vi "Rundenzeit.vi"(11 "Startlinie":bool) -> (3 "Rundenzeiten":dbl[](array[numeric])=[inf, inf, inf, inf, inf, inf, inf])   [LabVIEW 2016]
panel:
  # "Minimum"
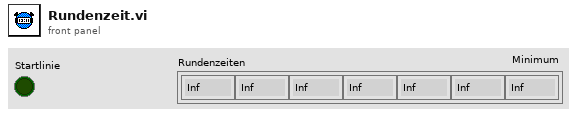
[diagram p1: front panel]
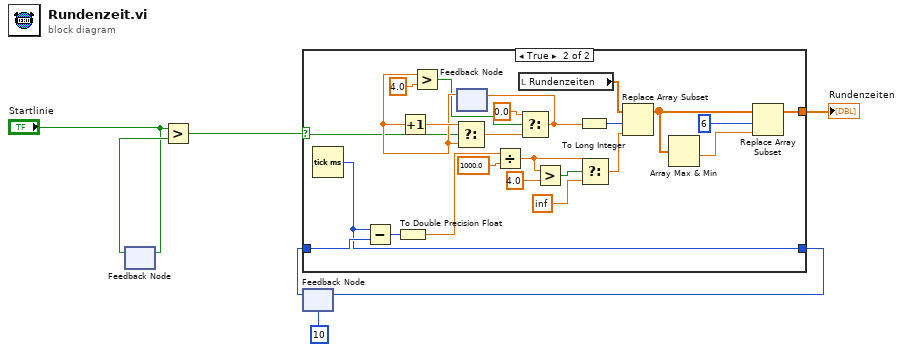
[diagram p0: block diagram]
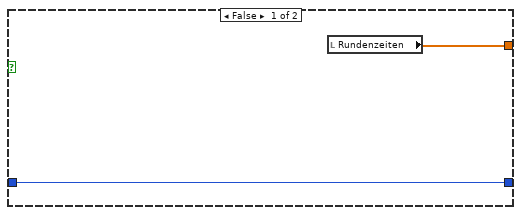
[diagram p2: hidden frame]
diagram:
  n1 = feedback #1() -> (w5:bool)  [unwired: 1 in]
  n2 = feedback-in #1("Startlinie") -> ()
  n3 = Greater?(x="Startlinie", y=w5) -> (0:w1:bool)
  n4 = feedback #2(u32 10 ("millisecond timer value")) -> (w6:u32)
  n5 = case shown="True" w1 {
    selector: w1 -> [_ w23]
    tunnel: [w9 w30] -> w7
    tunnel: w6 -> [w9 w33]
    tunnel: [w8 w19] -> w3
    frame False {
      n6 = local read "Rundenzeiten"() -> (w8:dbl[])
    }
    frame True {
      n7 = Tick Count (ms)() -> (millisecond timer value=w30:u32)
      n8 = Subtract(x=w30, y=w33) -> (x-y=w15:u32)
      n9 = To Double Precision Float(number=w15) -> (double precision float=w32:dbl)
      n10 = feedback #3() -> (w26:dbl)  [unwired: 1 in]
      n11 = Increment(x=w26) -> (x+1=w28:dbl)
      n12 = Greater?(x=w26, y=4.0) -> (0:w25:bool)
      n13 = Select(t=w28, s=w23, f=w26) -> (s? t:f=w27:dbl)
      n14 = Divide(x=w32, y=1000.0) -> (x/y=w12:dbl)
      n15 = local read "Rundenzeiten"() -> (w29:dbl[])
      n16 = Select(t=0.0, s=w25, f=w27) -> (s? t:f=w20:dbl)
      n17 = feedback-in #3(w20) -> ()
      n18 = Greater?(x=w12, y=4.0) -> (0:w13:bool)
      n19 = To Long Integer(number=w20) -> (32bit integer=w21:i32)
      n20 = Select(t=w12, s=w13, f=inf) -> (s? t:f=w11:dbl)
      n21 = Replace Array Subset(array=w29, new element=w11, index=w21) -> (w17:dbl[])
      n22 = Array Max & Min(array=w17) -> (min value=w16:dbl)  [unwired: 3 out]
      n23 = Replace Array Subset(array=w17, new element=w16, index=6) -> (w19:dbl[])
    }
  }
  "Rundenzeiten" <- w3
  n24 = feedback-in #2(w7) -> ()
